vi "DelayedTriggerFine.vi"(1 "Time Limit (us)":u32, 2 "Initiate":bool) -> (0 "Time Up":bool)   [LabVIEW 2019]
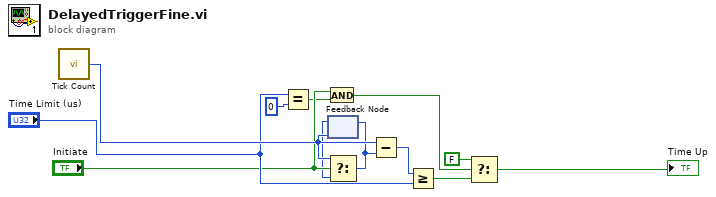
[diagram p0: block diagram]
diagram:
  n1 = call "Tick Count"() -> ("Tick Count(uSec)"=w12:u32)
  n2 = Equal?(x="Time Limit (us)", y=u32 0) -> (x = y?=w4:bool)
  n3 = And(x="Initiate", y=w4) -> (x .and. y?=w3:bool)
  n4 = feedback #1(w12) -> (w8:u32)
  n5 = Select(t=w12, s="Initiate", f=w8) -> (s? t:f=w7:u32)
  n6 = feedback-in #1(w7) -> ()
  n7 = Subtract(x=w12, y=w7) -> (x-y=w6:u32)
  n8 = Greater Or Equal?(x=w6, y="Time Limit (us)") -> (x >= y?=w1:bool)
  n9 = Select(t=FALSE, s=w3, f=w1) -> (s? t:f=→"Time Up":bool)
